vi "Get Method Name.vi"(8 "error in (no error)":errorcluster, 11 "Call in":refnum<class "Call.lvclass">) -> (0 "error out":errorcluster, 1 "Method Name":string, 2 "Object Name":string, 3 "Call out":refnum<class "Call.lvclass">)   [LabVIEW 2013, in "JKI_Python_Bridge_for_LV.lvlib" / "Call.lvclass"]
uses:
  Call.lvclass
  Call.lvclass/Call.ctl
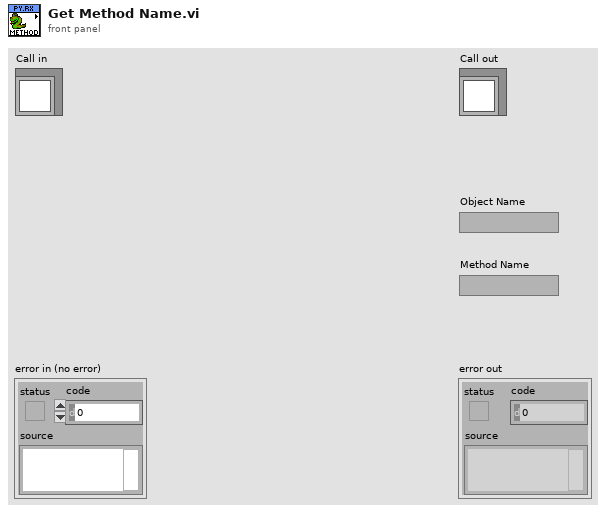
[diagram p1: front panel]
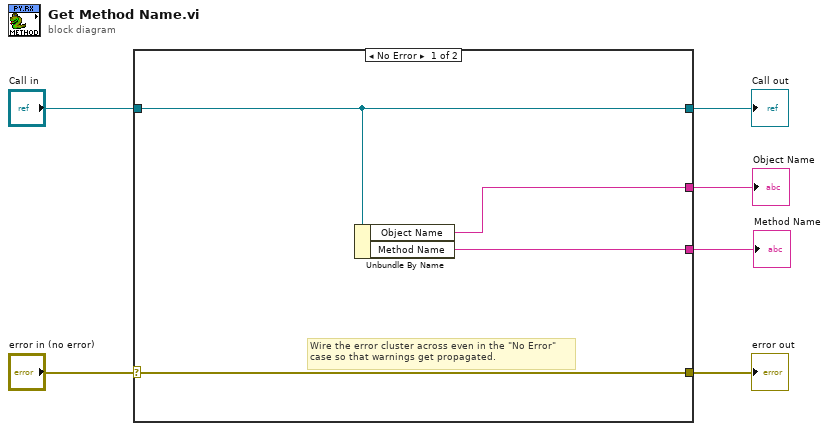
[diagram p0: block diagram]
diagram:
  n1 = case shown="No Error" "error in (no error)" {
    selector: "error in (no error)" -> [w10 w12]
    tunnel: [w10 w12] -> w5
    tunnel: [w9 w11] -> w3
    tunnel: "Call in" -> [w9 w11]
    tunnel: [w8 _] -> w2
    tunnel: [w7 _] -> w1
    frame No Error {
      # "Wire the error cluster across even in the \"No Error\"\ncase so that warnings get propagated."
      n2 = Unbundle By Name(w9) -> ("Object Name"=w7:string, "Method Name"=w8:string)
    }
    frame Error {
    }
  }
  "error out" <- w5
  "Call out" <- w3
  "Method Name" <- w2
  "Object Name" <- w1
